vi "switch.vi"(9 "Iterator":dbl, 10 "Numeric":dbl, 11 "Boolean":bool) -> (3 "Value":dbl)   [LabVIEW 2014]
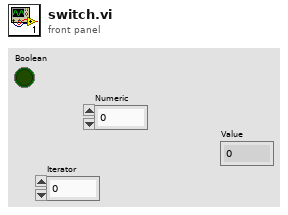
[diagram p1: front panel]
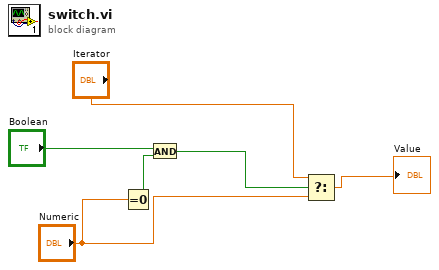
[diagram p0: block diagram]
diagram:
  n1 = Equal To 0?(x="Numeric") -> (x = 0?=w6:bool)
  n2 = And(x="Boolean", y=w6) -> (x .and. y?=w5:bool)
  n3 = Select(t="Iterator", s=w5, f="Numeric") -> (s? t:f=→"Value":dbl)
